vi "WB_correction_sub.vi"(3 "Input 2D":dbl[][](array[numeric])=[[0.0, 0.0, 0.0, 0.0, 0.0, 0.0, 0.0, 0.0, 0.0, 0.0, 0.0, 0.0, 0.0, 0.0, 0.0, 0.0, 0.0, 0.0, 0.0, 0.0, 0.0, 0.0, 0.0, 0.0, 0.0, 0.0, 0.0, 0.0, 0.0], [0.0, 0.0, 0.0, 0.0, 0.0, 0.0, 0.0, 0.0, 0.0, 0.0, 0.0, 0.0, 0.0, 0.0, 0.0, 0.0, 0.0, 0.0, 0.0, 0.0, 0.0, 0.0, 0.0, 0.0, 0.0, 0.0, 0.0, 0.0, 0.0], [0.0, 0.0, 0.0, 0.0, 0.0, 0.0, 0.0, 0.0, 0.0, 0.0, 0.0, 0.0, 0.0, 0.0, 0.0, 0.0, 0.0, 0.0, 0.0, 0.0, 0.0, 0.0, 0.0, 0.0, 0.0, 0.0, 0.0, 0.0, 0.0], [0.0, 0.0, 0.0, 0.0, 0.0, 0.0, 0.0, 0.0, 0.0, 0.0, 0.0, 0.0, 0.0, 0.0, 0.0, 0.0, 0.0, 0.0, 0.0, 0.0, 0.0, 0.0, 0.0, 0.0, 0.0, 0.0, 0.0, 0.0, 0.0], [0.0, 0.0, 0.0, 0.0, 0.0, 0.0, 0.0, 0.0, 0.0, 0.0, 0.0, 0.0, 0.0, 0.0, 0.0, 0.2, 0.6235294117647059, 0.9921568627450981, 0.6235294117647059, 0.19607843137254902, 0.0, 0.0, 0.0, 0.0, 0.0, 0.0, 0.0, 0.0, 0.0], [0.0, 0.0, 0.0, 0.0, 0.0, 0.0, 0.0, 0.0, 0.0, 0.0, 0.0, 0.0, 0.0, 0.0, 0.18823529411764706, 0.9333333333333333, 0.9882352941176471, 0.9882352941176471, 0.9882352941176471, 0.9294117647058824, 0.0, 0.0, 0.0, 0.0, 0.0, 0.0, 0.0, 0.0, 0.0], [0.0, 0.0, 0.0, 0.0, 0.0, 0.0, 0.0, 0.0, 0.0, 0.0, 0.0, 0.0, 0.0, 0.21176470588235294, 0.8901960784313725, 0.9921568627450981, 0.9882352941176471, 0.9372549019607843, 0.9137254901960784, 0.9882352941176471, 0.2235294117647059, 0.023529411764705882, 0.0, 0.0, 0.0, 0.0, 0.0, 0.0, 0.0], [0.0, 0.0, 0.0, 0.0, 0.0, 0.0, 0.0, 0.0, 0.0, 0.0, 0.0, 0.0392156862745098, 0.23529411764705882, 0.8784313725490196, 0.9882352941176471, 0.9921568627450981, 0.9882352941176471, 0.792156862745098, 0.32941176470588235, 0.9882352941176471, 0.9921568627450981, 0.47843137254901963, 0.0, 0.0, 0.0, 0.0, 0.0, 0.0, 0.0], [0.0, 0.0, 0.0, 0.0, 0.0, 0.0, 0.0, 0.0, 0.0, 0.0, 0.0, 0.6392156862745098, 0.9882352941176471, 0.9882352941176471, 0.9882352941176471, 0.9921568627450981, 0.9882352941176471, 0.9882352941176471, 0.3764705882352941, 0.7411764705882353, 0.9921568627450981, 0.6549019607843137, 0.0, 0.0, 0.0, 0.0, 0.0, 0.0, 0.0], [0.0, 0.0, 0.0, 0.0, 0.0, 0.0, 0.0, 0.0, 0.0, 0.0, 0.2, 0.9333333333333333, 0.9921568627450981, 0.9921568627450981, 0.7450980392156863, 0.4470588235294118, 0.9921568627450981, 0.8941176470588236, 0.1843137254901961, 0.30980392156862746, 1.0, 0.6588235294117647, 0.0, 0.0, 0.0, 0.0, 0.0, 0.0, 0.0], [0.0, 0.0, 0.0, 0.0, 0.0, 0.0, 0.0, 0.0, 0.0, 0.18823529411764706, 0.9333333333333333, 0.9882352941176471, 0.9882352941176471, 0.7019607843137254, 0.047058823529411764, 0.29411764705882354, 0.4745098039215686, 0.08235294117647059, 0.0, 0.0, 0.9921568627450981, 0.9529411764705882, 0.19607843137254902, 0.0, 0.0, 0.0, 0.0, 0.0, 0.0], [0.0, 0.0, 0.0, 0.0, 0.0, 0.0, 0.0, 0.0, 0.14901960784313725, 0.6470588235294118, 0.9921568627450981, 0.9137254901960784, 0.8156862745098039, 0.32941176470588235, 0.0, 0.0, 0.0, 0.0, 0.0, 0.0, 0.9921568627450981, 0.9882352941176471, 0.6470588235294118, 0.0, 0.0, 0.0, 0.0, 0.0, 0.0], [0.0, 0.0, 0.0, 0.0, 0.0, 0.0, 0.0, 0.027450980392156862, 0.6980392156862745, 0.9882352941176471, 0.9411764705882353, 0.2784313725490196, 0.07450980392156863, 0.10980392156862745, 0.0, 0.0, 0.0, 0.0, 0.0, 0.0, 0.9921568627450981, 0.9882352941176471, 0.7647058823529411, 0.0, 0.0, 0.0, 0.0, 0.0, 0.0], [0.0, 0.0, 0.0, 0.0, 0.0, 0.0, 0.0, 0.2235294117647059, 0.9882352941176471, 0.9882352941176471, 0.24705882352941178, 0.0, 0.0, 0.0, 0.0, 0.0, 0.0, 0.0, 0.0, 0.0, 0.9921568627450981, 0.9882352941176471, 0.7647058823529411, 0.0, 0.0, 0.0, 0.0, 0.0, 0.0], [0.0, 0.0, 0.0, 0.0, 0.0, 0.0, 0.0, 0.7764705882352941, 0.9921568627450981, 0.7450980392156863, 0.0, 0.0, 0.0, 0.0, 0.0, 0.0, 0.0, 0.0, 0.0, 0.0, 1.0, 0.9921568627450981, 0.7686274509803922, 0.0, 0.0, 0.0, 0.0, 0.0, 0.0], [0.0, 0.0, 0.0, 0.0, 0.0, 0.0, 0.2980392156862745, 0.9647058823529412, 0.9882352941176471, 0.4392156862745098, 0.0, 0.0, 0.0, 0.0, 0.0, 0.0, 0.0, 0.0, 0.0, 0.0, 0.9921568627450981, 0.9882352941176471, 0.5803921568627451, 0.0, 0.0, 0.0, 0.0, 0.0, 0.0], [0.0, 0.0, 0.0, 0.0, 0.0, 0.0, 0.3333333333333333, 0.9882352941176471, 0.9019607843137255, 0.09803921568627451, 0.0, 0.0, 0.0, 0.0, 0.0, 0.0, 0.0, 0.0, 0.027450980392156862, 0.5294117647058824, 0.9921568627450981, 0.7294117647058823, 0.047058823529411764, 0.0, 0.0, 0.0, 0.0, 0.0, 0.0], [0.0, 0.0, 0.0, 0.0, 0.0, 0.0, 0.3333333333333333, 0.9882352941176471, 0.8745098039215686, 0.0, 0.0, 0.0, 0.0, 0.0, 0.0, 0.0, 0.0, 0.027450980392156862, 0.5137254901960784, 0.9882352941176471, 0.8823529411764706, 0.2784313725490196, 0.0, 0.0, 0.0, 0.0, 0.0, 0.0, 0.0], [0.0, 0.0, 0.0, 0.0, 0.0, 0.0, 0.3333333333333333, 0.9882352941176471, 0.5686274509803921, 0.0, 0.0, 0.0, 0.0, 0.0, 0.0, 0.0, 0.18823529411764706, 0.6470588235294118, 0.9882352941176471, 0.6784313725490196, 0.0, 0.0, 0.0, 0.0, 0.0, 0.0, 0.0, 0.0, 0.0], [0.0, 0.0, 0.0, 0.0, 0.0, 0.0, 0.33725490196078434, 0.9921568627450981, 0.8823529411764706, 0.0, 0.0, 0.0, 0.0, 0.0, 0.0, 0.4470588235294118, 0.9333333333333333, 0.9921568627450981, 0.6352941176470588, 0.0, 0.0, 0.0, 0.0, 0.0, 0.0, 0.0, 0.0, 0.0, 0.0], [0.0, 0.0, 0.0, 0.0, 0.0, 0.0, 0.3333333333333333, 0.9882352941176471, 0.9764705882352941, 0.5725490196078431, 0.18823529411764706, 0.11372549019607843, 0.3333333333333333, 0.6980392156862745, 0.8823529411764706, 0.9921568627450981, 0.8745098039215686, 0.6549019607843137, 0.2196078431372549, 0.0, 0.0, 0.0, 0.0, 0.0, 0.0, 0.0, 0.0, 0.0, 0.0], [0.0, 0.0, 0.0, 0.0, 0.0, 0.0, 0.3333333333333333, 0.9882352941176471, 0.9882352941176471, 0.9882352941176471, 0.8980392156862745, 0.8431372549019608, 0.9882352941176471, 0.9882352941176471, 0.9882352941176471, 0.7686274509803922, 0.5098039215686274, 0.0, 0.0, 0.0, 0.0, 0.0, 0.0, 0.0, 0.0, 0.0, 0.0, 0.0, 0.0], [0.0, 0.0, 0.0, 0.0, 0.0, 0.0, 0.10980392156862745, 0.7803921568627451, 0.9882352941176471, 0.9882352941176471, 0.9921568627450981, 0.9882352941176471, 0.9882352941176471, 0.9137254901960784, 0.5686274509803921, 0.0, 0.0, 0.0, 0.0, 0.0, 0.0, 0.0, 0.0, 0.0, 0.0, 0.0, 0.0, 0.0, 0.0], [0.0, 0.0, 0.0, 0.0, 0.0, 0.0, 0.0, 0.09803921568627451, 0.5019607843137255, 0.9882352941176471, 0.9921568627450981, 0.9882352941176471, 0.5529411764705883, 0.1450980392156863, 0.0, 0.0, 0.0, 0.0, 0.0, 0.0, 0.0, 0.0, 0.0, 0.0, 0.0, 0.0, 0.0, 0.0, 0.0], [0.0, 0.0, 0.0, 0.0, 0.0, 0.0, 0.0, 0.0, 0.0, 0.0, 0.0, 0.0, 0.0, 0.0, 0.0, 0.0, 0.0, 0.0, 0.0, 0.0, 0.0, 0.0, 0.0, 0.0, 0.0, 0.0, 0.0, 0.0, 0.0], [0.0, 0.0, 0.0, 0.0, 0.0, 0.0, 0.0, 0.0, 0.0, 0.0, 0.0, 0.0, 0.0, 0.0, 0.0, 0.0, 0.0, 0.0, 0.0, 0.0, 0.0, 0.0, 0.0, 0.0, 0.0, 0.0, 0.0, 0.0, 0.0], [0.0, 0.0, 0.0, 0.0, 0.0, 0.0, 0.0, 0.0, 0.0, 0.0, 0.0, 0.0, 0.0, 0.0, 0.0, 0.0, 0.0, 0.0, 0.0, 0.0, 0.0, 0.0, 0.0, 0.0, 0.0, 0.0, 0.0, 0.0, 0.0], [0.0, 0.0, 0.0, 0.0, 0.0, 0.0, 0.0, 0.0, 0.0, 0.0, 0.0, 0.0, 0.0, 0.0, 0.0, 0.0, 0.0, 0.0, 0.0, 0.0, 0.0, 0.0, 0.0, 0.0, 0.0, 0.0, 0.0, 0.0, 0.0]]) -> (1 "Output 2D 2":dbl[][](array[numeric]))   [LabVIEW 2021]
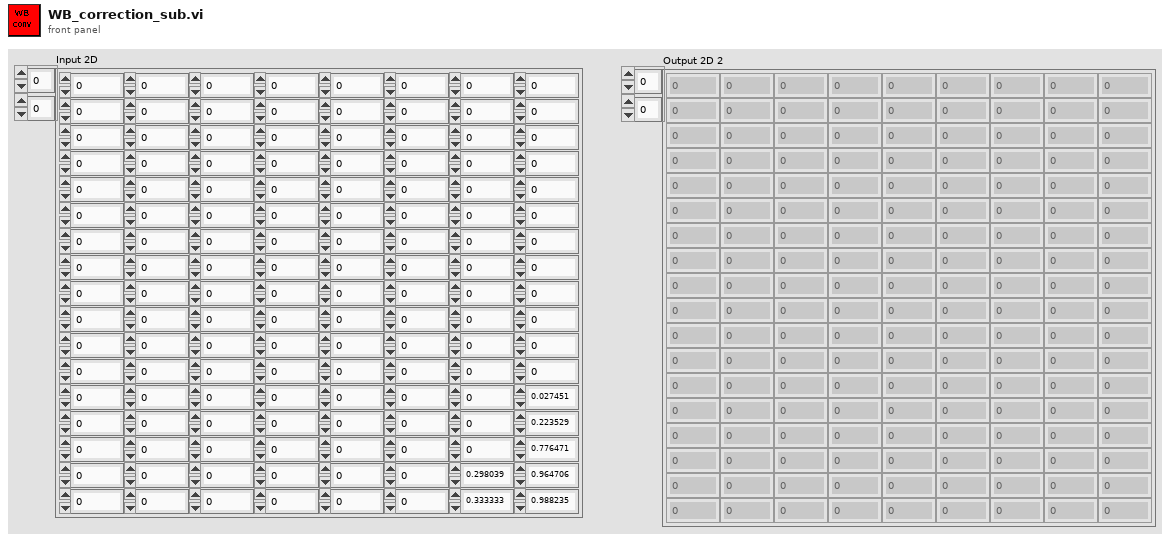
[diagram p1: front panel]
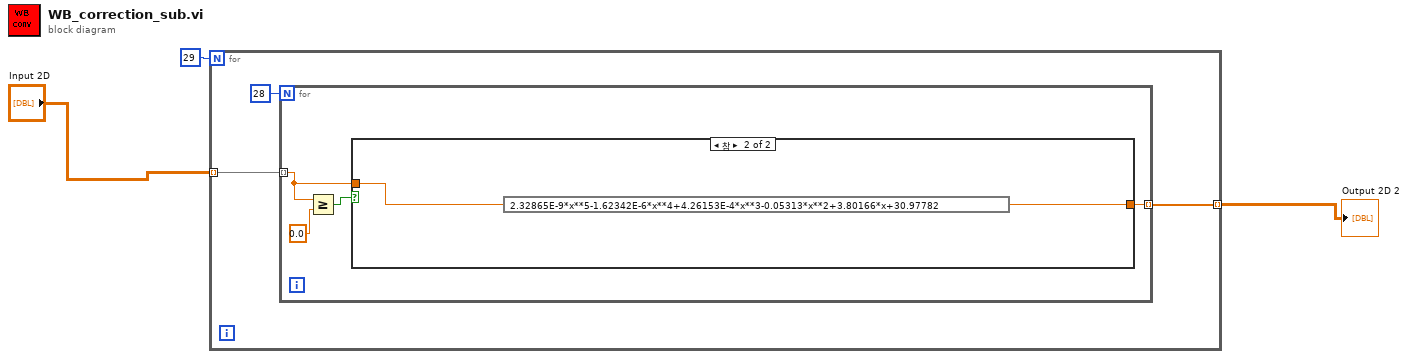
[diagram p0: block diagram]
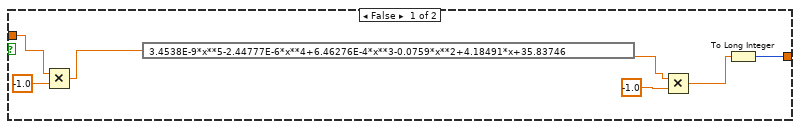
[diagram p2: hidden frame]
diagram:
  n1 = for {
    N: 29 -> [_]
    tunnel: "Input 2D" -> [w5] mode=indexing
    tunnel: [w4] -> w2 mode=indexing
    n2 = for {
      N: 28 -> [_]
      tunnel: w5 -> [w8] mode=indexing
      tunnel: [w7] -> w4 mode=indexing
      n3 = Greater Or Equal?(x=w8, y=0.0) -> (x >= y?=w10:bool)
      n4 = case shown="참" w10 {
        tunnel: w8 -> [w17 w19]
        tunnel: [w11 w18] -> w7
        frame False {
          n5 = Multiply(x=w17, y=-1.0) -> (x*y=w15:dbl)
          n6 = expression code="3.4538E-9*x**5-2.44777E-6*x**4+6.46276E-4*x**3-0.0759*x**2+4.18491*x+35.83746"(w15) -> (w13:dbl)
          n7 = Multiply(x=w13, y=-1.0) -> (x*y=w12:dbl)
          n8 = To Long Integer(number=w12) -> (32bit integer=w11:i32)
        }
        frame True {
          n9 = expression code="2.32865E-9*x**5-1.62342E-6*x**4+4.26153E-4*x**3-0.05313*x**2+3.80166*x+30.97782"(w19) -> (w18:dbl)
        }
      }
    }
  }
  "Output 2D 2" <- w2
